vi "FrameShiftCorrect.vi"(4 "bytes streaming per frame":u16, 7 "U16Data":u16[](array[numeric])) -> (0 "MatchFound":bool, 1 "NumRemaining":i32, 2 "NumElementsOut":i32, 3 "binarydataShifted":u16[](array[numeric]))   [LabVIEW 2017]
doc: "VI tries to correct frame shifts/misreads in streaming Intsy Data. Shifting ID is based on data frame format always starting and ending with pre-defined characters ('I' and magic num). \n\nInputs: U16 data array\n\nOutputs: frame shifted array that terminates after last full frame read\nRemaining array: trailing elements left over"
panel:
  out "leftoverelements":u16[](array[numeric])
  out "fragmentedFrame":bool
  out "NoMatch":bool
  out "NumElemInit":i32
  out "iter":i32
  out "indexMagicnum":i32
  in  "macignum":u16=8481
  out "indexI":i32
  in  "Ichar":u16=73
  out "wordsperframe":i16
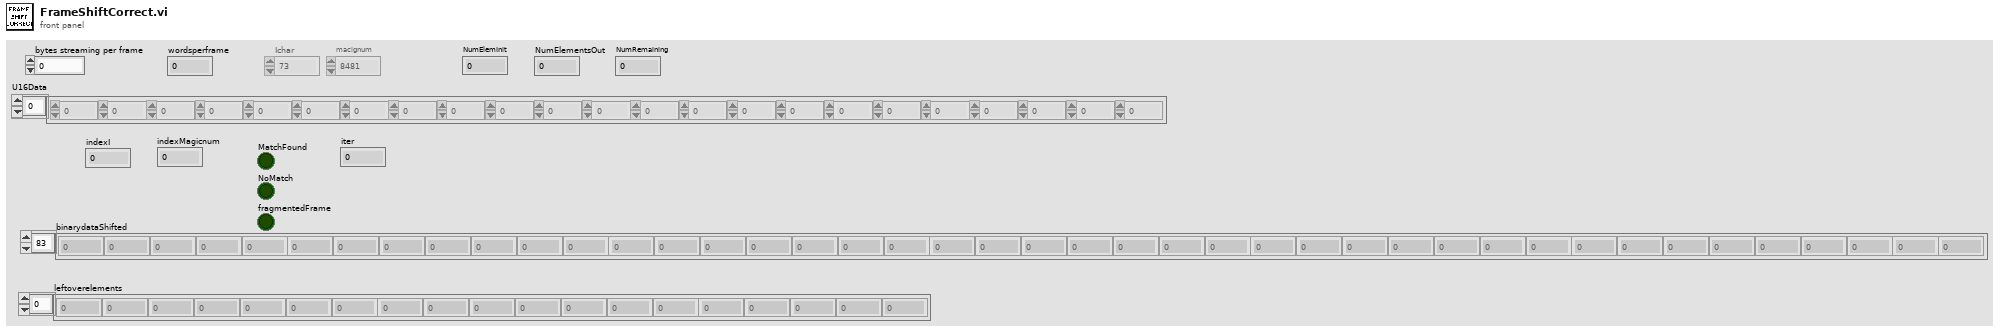
[diagram p1: front panel]
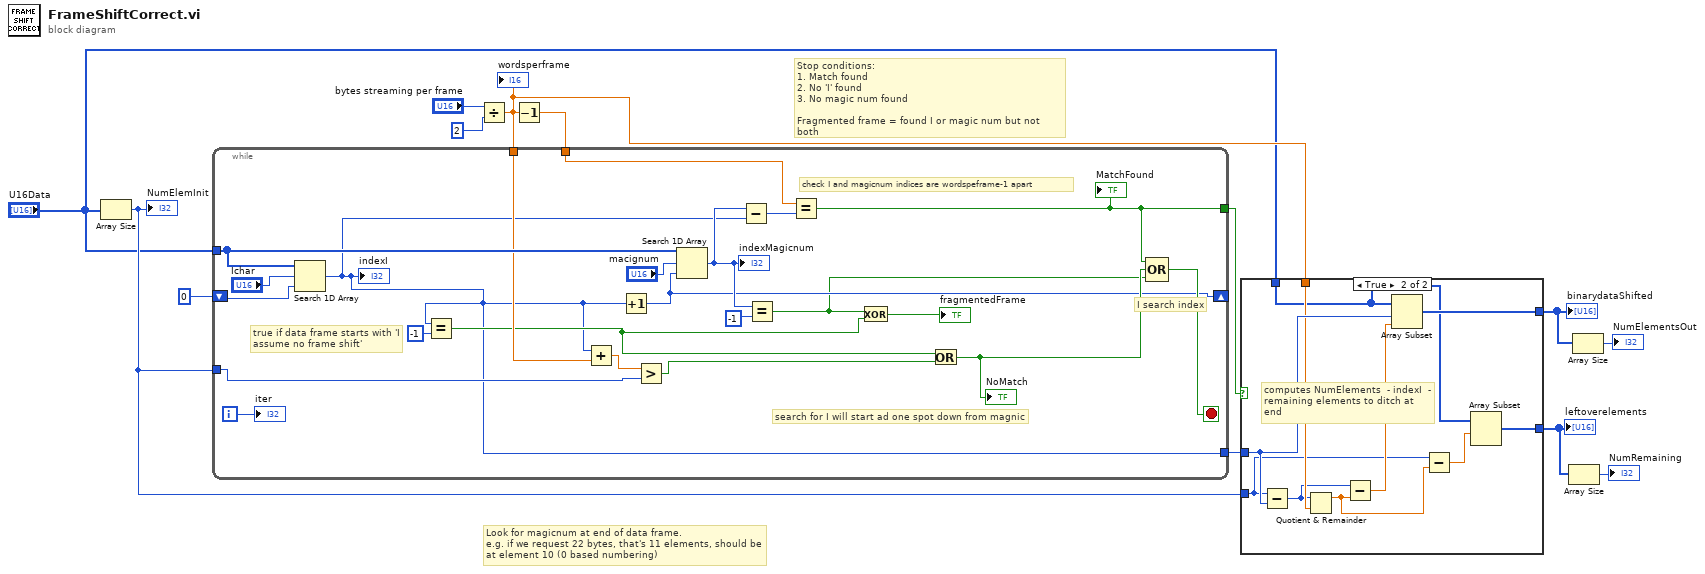
[diagram p0: block diagram]
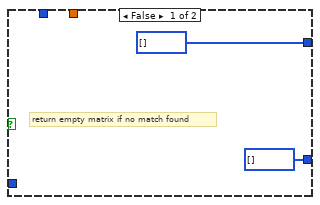
[diagram p2: hidden frame]
diagram:
  # "Stop conditions:\n1. Match found\n2. No 'I' found\n3. No magic num found\n\nFragmented frame = found I or magic num but not both"
  # "Look for magicnum at end of data frame.\ne.g. if we request 22 bytes, that's 11 elements, should be\nat element 10 (0 based numbering)"
  n1 = Array Size(array="U16Data") -> (size(s)=w9:i32)
  "NumElemInit" <- w9
  n2 = Divide(x="bytes streaming per frame", y=u16 2) -> (x/y=w7:dbl)
  "wordsperframe" <- w7
  n3 = Decrement(x=w7) -> (x-1=w11:dbl)
  n4 = while {
    tunnel: w11 -> [w33]
    shift-right: [w17] -> _
    shift-left: u16 0 ("y") -> [w31]
    tunnel: "U16Data" -> [w29]
    tunnel: w9 -> [w26]
    tunnel: w7 -> [w24]
    tunnel: [w15] -> w8
    tunnel: [w14] -> w6
    i -> [w30]
    stop <- w27 stop-if-true
    # "I search index"
    # "check I and magicnum indices are wordspeframe-1 apart"
    # "search for I will start ad one spot down from magnic"
    # "true if data frame starts with 'I\nassume no frame shift'"
    n5 = Search 1D Array(1D array=w29, element="Ichar", start index (0)=w31) -> (index of element=w15:i32)
    "indexI" <- w15
    n6 = Equal?(x=w15, y=-1) -> (x = y?=w19:bool)
    n7 = Add(x=w15, y=w24) -> (x+y=w25:dbl)
    n8 = Increment(x=w15) -> (x+1=w17:i32)
    n9 = Greater?(x=w25, y=w26) -> (0:w23:bool)
    n10 = Search 1D Array(1D array=w29, element="macignum", start index (0)=w17) -> (index of element=w21:i32)
    "indexMagicnum" <- w21
    n11 = Subtract(x=w21, y=w15) -> (x-y=w32:i32)
    n12 = Equal?(x=w21, y=-1) -> (x = y?=w16:bool)
    n13 = Equal?(x=w33, y=w32) -> (x = y?=w14:bool)
    "MatchFound" <- w14
    n14 = Exclusive Or(1:w19, 2:w16) -> (0:→"fragmentedFrame":bool)
    n15 = Or(x=w19, y=w23) -> (x .or. y?=w22:bool)
    "NoMatch" <- w22
    n16 = Compound Arithmetic op=OR(w14, w22, w16) -> (w27:bool)
    "iter" <- w30
  }
  n17 = case shown="True" w6 {
    tunnel: "U16Data" -> [_ w42]
    tunnel: w9 -> [_ w40]
    tunnel: w8 -> [_ w47]
    tunnel: w7 -> [_ w46]
    tunnel: [u16[] [] w43] -> w4
    tunnel: [u16[] [] w38] -> w3
    frame False {
      # "return empty matrix if no match found"
    }
    frame True {
      # "computes NumElements  - indexI  - remaining elements to ditch at end"
      n18 = Subtract(x=w40, y=w47) -> (x-y=w45:i32)
      n19 = Quotient & Remainder(x=w45, y=w46) -> (x-y*floor(x/y)=w39:dbl)  [unwired: 1 out]
      n20 = Subtract(x=w45, y=w39) -> (x-y=w44:dbl)
      n21 = Array Subset(array=w42, index=w47, length=w44) -> (w43:u16[])
      n22 = Subtract(x=w40, y=w39) -> (x-y=w41:dbl)
      n23 = Array Subset(array=w42, index=w41) -> (w38:u16[])  [unwired: 1 in]
    }
  }
  "binarydataShifted" <- w4
  "leftoverelements" <- w3
  n24 = Array Size(array=w3) -> (size(s)=→"NumRemaining":i32)
  n25 = Array Size(array=w4) -> (size(s)=→"NumElementsOut":i32)
